vi "Milestone4Testing.vi"() -> ()   [LabVIEW 2014]
uses:
  Controls/Direction enum.ctl
panel:
  out "X Guess S2":i32
  in  "stop 2":bool
  out "X guess":i32
  in  "stop":bool
  out "Angle stage 1 end":T1 items=["0", "45", "90", "135", "180", "225", "270", "315"]
  in  "Angle":T1 items=["0", "45", "90", "135", "180", "225", "270", "315"]
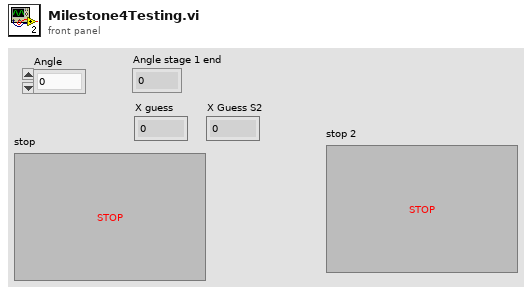
[diagram p1: front panel]
types:
  T1 = typedef "Direction enum.ctl" = u16
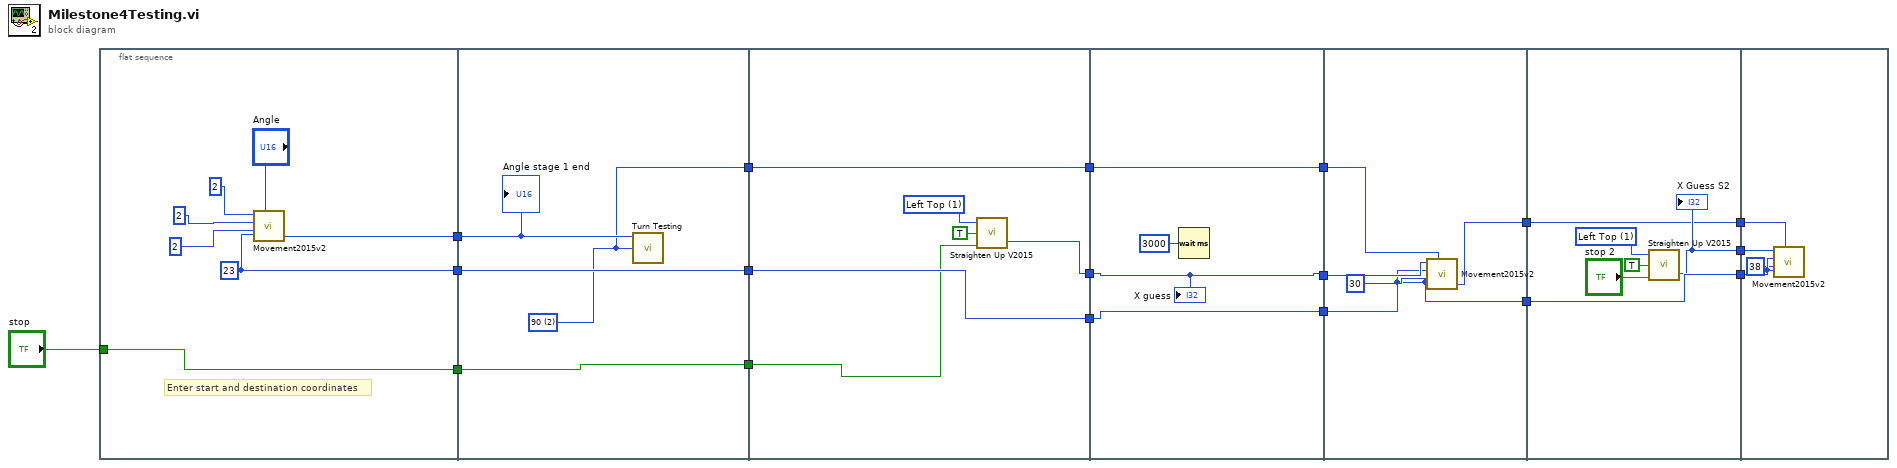
[diagram p0: block diagram]
diagram:
  n1 = flat-sequence {
    tunnel: [w21] -> w18
    tunnel: [w20] -> w16
    tunnel: [w19] -> w2
    tunnel: "stop" -> [w19]
    tunnel: w18 -> [w29]
    tunnel: w16 -> [w28]
    tunnel: [w28] -> w5
    tunnel: [w27] -> w4
    tunnel: [w26] -> w3
    tunnel: w2 -> [w26]
    tunnel: [w33] -> w15
    tunnel: [w32] -> w13
    tunnel: [w31] -> w11
    tunnel: w4 -> [w31]
    tunnel: w5 -> [w33]
    tunnel: w3 -> [w30]
    tunnel: [w38] -> w17
    tunnel: w15 -> [w37]
    tunnel: [w37] -> w14
    tunnel: w13 -> [w38]
    tunnel: [w36] -> w12
    tunnel: w11 -> [w36]
    tunnel: w17 -> [w44]
    tunnel: w14 -> [w41]
    tunnel: w12 -> [w42]
    tunnel: [w41] -> w9
    tunnel: [w40] -> w7
    tunnel: [w47] -> w10
    tunnel: w9 -> [w47]
    tunnel: [w46] -> w8
    tunnel: w7 -> [w45]
    tunnel: [w45] -> w6
    tunnel: w10 -> [w54]
    tunnel: w8 -> [w52]
    tunnel: w6 -> [w51]
    frame #0 {
      w20 = i16 23 ("Destination Y")
      # "Enter start and destination coordinates"
      n2 = call "Movement2015v2.vi"("Start X"=i16 2, "Angle"="Angle", "Start Y"=i16 2, "Destination X"=i16 2, "Destination Y"=w20) -> ("Angle out 2"=w21:T1)  [unwired: 3 in]
    }
    frame #1 {
      w27 = T1 2 items=["0", "45", "90", "135", "180", "225", "270", "315"] ("end angle")
      n3 = call "Turn Testing.vi"("end angle"=w27, "start angle"=w29) -> ()  [unwired: 3 in, 1 out]
      "Angle stage 1 end" <- w29
    }
    frame #2 {
      w34 = u16 1 items=["Center Top", "Left Top", "Center Bottom", "Right Bottom", "Home", "Right mid", "Center Top 0", "Panting rowe"] ("Estimated Location")
      n4 = call "Straighten Up V2015.vi"("stop"=w30, "10CM?"=TRUE, "Estimated Location"=w34) -> ("X Guess"=w32:i32)  [unwired: 1 out]
    }
    frame #3 {
      n5 = Wait (ms)(milliseconds to wait=u32 3000) -> ()  [unwired: 1 out]
      "X guess" <- w38
    }
    frame #4 {
      n6 = call "Movement2015v2.vi"("Start X"=w44, "Angle"=w42, "Start Y"=w41, "Destination X"=i16 30, "Destination Y"=w41) -> ("Angle out 2"=w40:T1)  [unwired: 3 in]
    }
    frame #5 {
      w49 = u16 1 items=["Center Top", "Left Top", "Center Bottom", "Right Bottom", "Home", "Right mid", "Center Top 0", "Panting rowe"] ("Estimated Location")
      n7 = call "Straighten Up V2015.vi"("stop"="stop 2", "10CM?"=TRUE, "Estimated Location"=w49) -> ("X Guess"=w46:i32)  [unwired: 1 out]
      "X Guess S2" <- w46
    }
    frame #6 {
      n8 = call "Movement2015v2.vi"("Start X"=w52, "Angle"=w51, "Start Y"=w54, "Destination X"=i16 38, "Destination Y"=w54) -> ()  [unwired: 3 in, 1 out]
    }
  }
